vi "Configure Channel.vi"(0 "VISA resource name":refnum<visa-resource-name>, 1 "Enable Channel (T: Enable)":bool=TRUE, 5 "Channel (0: Channel 1)":u16(ring) items=["Channel 1", "Channel 2", "Channel 3", "Channel 4"], 7 "Vertical Coupling (0: AC)":u16(ring) items=["AC", "DC"], 9 "Probe Attenuation (10.0)":dbl=10.0, 11 "error in (no error)":errorcluster, 12 "Vertical Range (10.0 V)":dbl=10.0, 13 "Vertical Offset (0.0 V)":dbl) -> (4 "VISA resource name out":refnum<visa-resource-name>, 15 "error out":errorcluster)   [LabVIEW 2017, in "Agilent 6000 Series.lvlib"]
doc: "Configures the common properties of the oscilloscope's vertical subsystem for the specified channel. Call this VI for each channel you want to enable to acquire waveforms.\n\nNote:\nThe channel settings will not be applied if the channel is not enabled."
uses:
  <instrlib>/Agilent 6000 Series/Agilent 6000 Series.lvlib
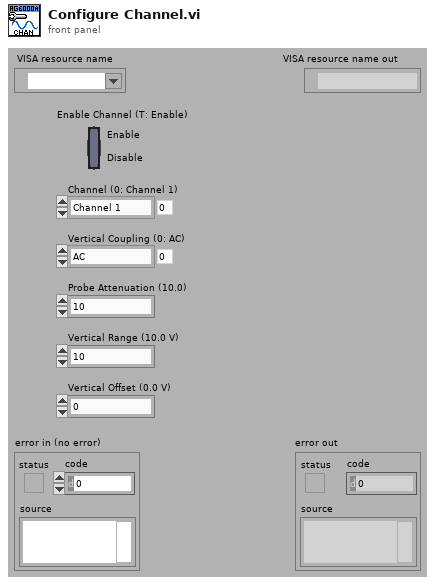
[diagram p1: front panel]
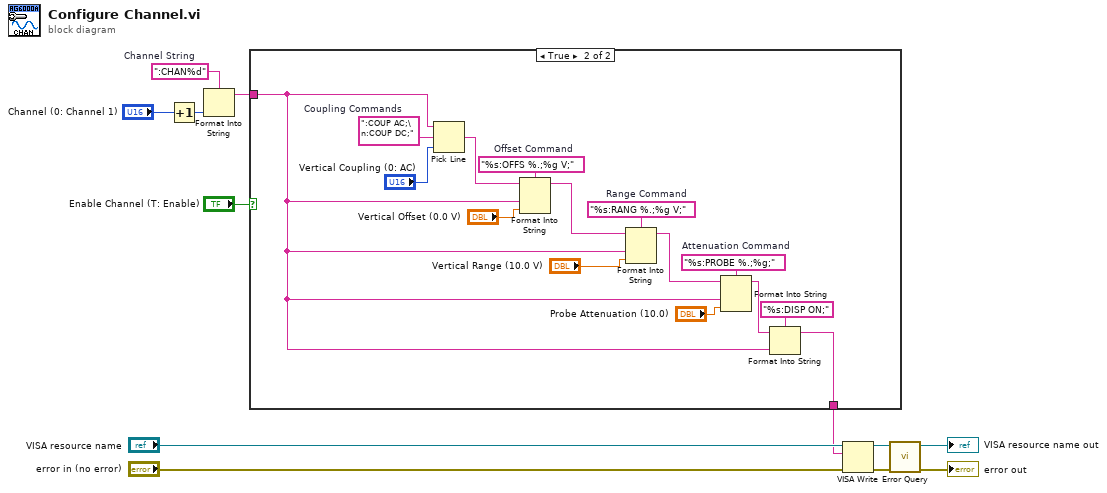
[diagram p0: block diagram]
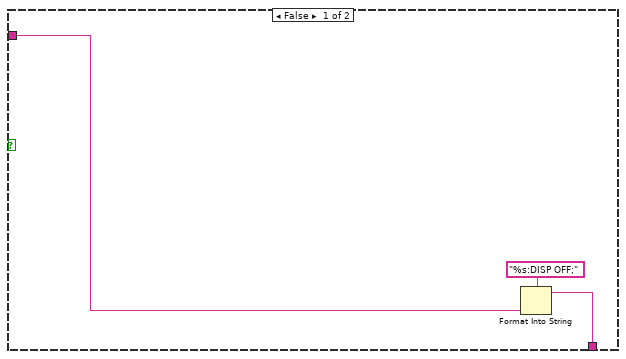
[diagram p2: hidden frame]
diagram:
  w4 = ":CHAN%d"  # Channel String
  n1 = Increment(x="Channel (0: Channel 1)") -> (x+1=w2:u16)
  n2 = Format Into String(format string=w4, w2) -> (resulting string=w3:string)  [unwired: 2 in, 1 out]
  n3 = case shown="True" "Enable Channel (T: Enable)" {
    tunnel: [w13 w19] -> w6
    tunnel: w3 -> [w14 w16]
    frame False {
      n4 = Format Into String(format string="%s:DISP OFF;", w14) -> (resulting string=w13:string)  [unwired: 2 in, 1 out]
    }
    frame True {
      w25 = "%s:PROBE %.;%g;"  # Attenuation Command
      w26 = "%s:RANG %.;%g V;"  # Range Command
      w28 = "%s:OFFS %.;%g V;"  # Offset Command
      w30 = ":COUP AC;\n:COUP DC;"  # Coupling Commands
      n5 = Pick Line(string ("")=w16, multi-line string=w30, line index="Vertical Coupling (0: AC)") -> (output string=w18:string)
      n6 = Format Into String(format string=w28, initial string=w18, w16, "Vertical Offset (0.0 V)") -> (resulting string=w17:string)  [unwired: 1 in, 1 out]
      n7 = Format Into String(format string=w26, initial string=w17, w16, "Vertical Range (10.0 V)") -> (resulting string=w22:string)  [unwired: 1 in, 1 out]
      n8 = Format Into String(format string=w25, initial string=w22, w16, "Probe Attenuation (10.0)") -> (resulting string=w20:string)  [unwired: 1 in, 1 out]
      n9 = Format Into String(format string="%s:DISP ON;", initial string=w20, w16) -> (resulting string=w19:string)  [unwired: 1 in, 1 out]
    }
  }
  n10 = VISA Write(VISA resource name="VISA resource name", write buffer=w6, error in (no error)="error in (no error)") -> (VISA resource name out=w8:refnum<visa-resource-name>, error out=w7:errorcluster)  [unwired: 1 out]
  n11 = call <instrlib>:"Error Query.vi"("error in (no error)"=w7, "VISA resource name"=w8) -> ("error out"=→"error out":errorcluster, "VISA resource name out"=→"VISA resource name out":refnum<visa-resource-name>)  [unwired: 6 in, 2 out]
